vi "ChannelType_2D-Array-CDB.vi"(9 "error in":errorcluster, 11 "Array in":cdb[][](array[numeric])) -> (1 "error out":errorcluster, 2 "ChannelType":dbl, 3 "Array out":cdb[][](array[numeric]))   [LabVIEW 2020, in "OpenLvVision_OpenCv.lvlib"]
uses:
  OpenLvVision_OpenCv.lvlib
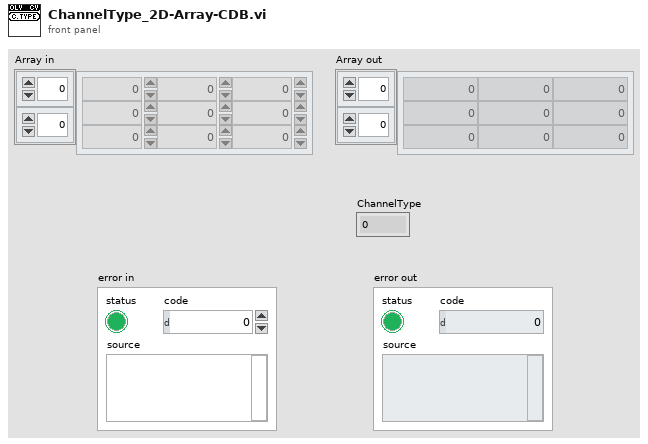
[diagram p1: front panel]
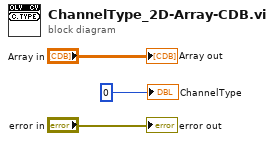
[diagram p0: block diagram]
diagram:
  "error out" <- "error in"
  "Array out" <- "Array in"
  "ChannelType" <- u16 0
